vi "SmartMotor_SendCommand - single motor.vi"(0 "VISA In":refnum<visa-resource-name>, 1 "MotorCmd":T4, 2 "Set ModeSelect":T3, 5 "Adhoc Input":T2, 7 "MotorSpecifier(M1)":T1=enum."M1", 9 "ReadWait":u32=50, 11 "error in":errorcluster, 12 "NumericInput":dbl caption="Set Encoder Value(cnts)", 13 "BooleanInput":bool) -> (4 "VISA Out":refnum<visa-resource-name>, 6 "Response Str":string, 8 "Cmd Str out":string, 15 "error out":errorcluster)   [LabVIEW 2020]
doc: "Developed by Kevin Thompson\nkevin@thompsonengineering.net\n\nCopyright 2018-2020\nThompson Engineering, LLC"
uses:
  TD MotorCommands - single motor--enum.ctl
  TD MotorModeSelect_enum.ctl
  TD SerialBusMotorSpecifier_enum.ctl
panel:
  # "Unlisted Command"
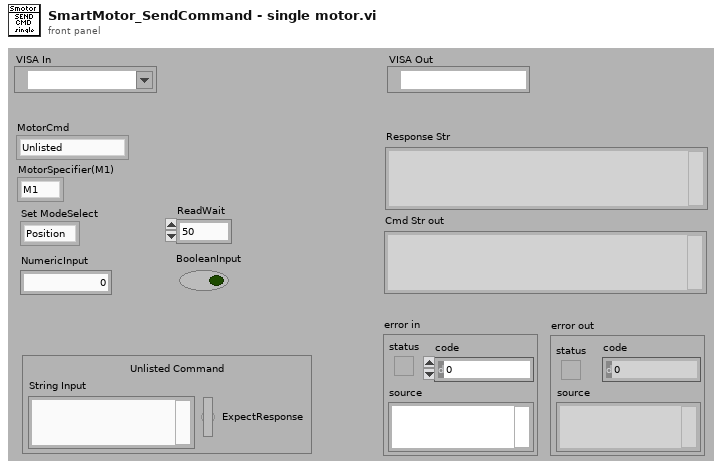
[diagram p1: front panel]
types:
  T1 = typedef "TD SerialBusMotorSpecifier_enum.ctl" = enum16{"None", "Global", "M1", "M2", "M3"}
  T2 = cluster{"String Input":string, "ExpectResponse":bool}
  T3 = typedef "TD MotorModeSelect_enum.ctl" = enum16{"Position", "Velocity", "Torque"}
  T4 = typedef "TD MotorCommands - single motor--enum.ctl" = enum16{"Unlisted", "AbortMotion", "StopMotion", "DisableMotor", "ClearErrors", "ZeroEncoder", "SetMode", "GO", "SetEncoder", "En/Ds LmtSwitchs"}
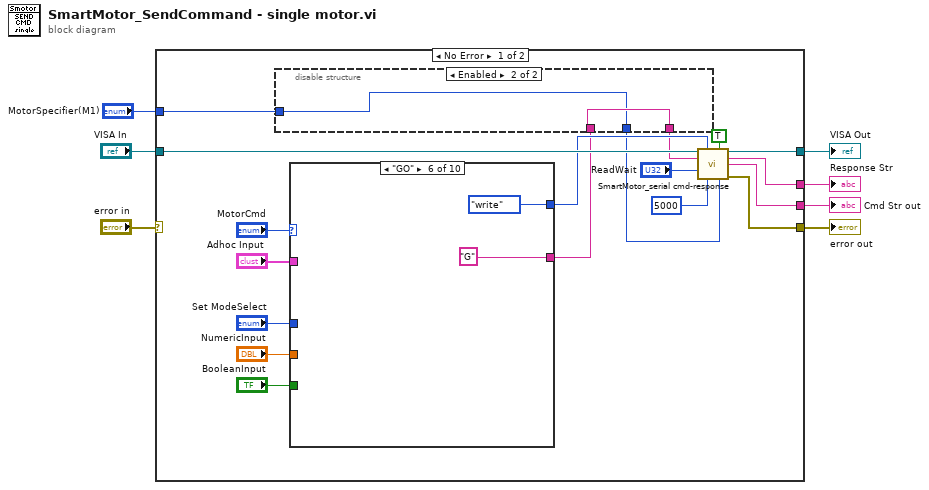
[diagram p0: block diagram]
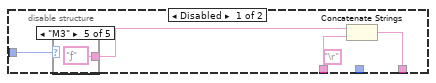
[diagram p2: hidden frame]
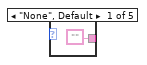
[diagram p3: hidden frame]
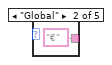
[diagram p4: hidden frame]
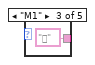
[diagram p5: hidden frame]
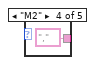
[diagram p6: hidden frame]
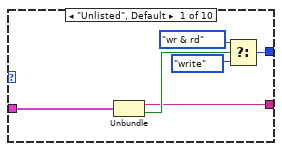
[diagram p7: hidden frame]
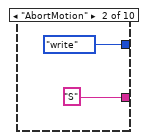
[diagram p8: hidden frame]
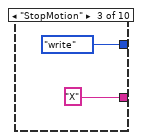
[diagram p9: hidden frame]
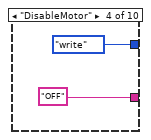
[diagram p10: hidden frame]
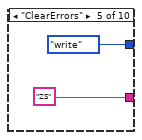
[diagram p11: hidden frame]
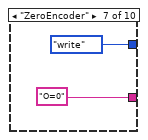
[diagram p12: hidden frame]
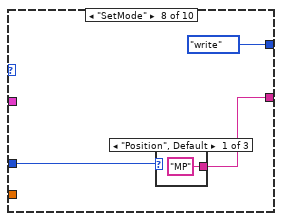
[diagram p13: hidden frame]
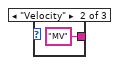
[diagram p14: hidden frame]
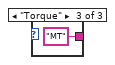
[diagram p15: hidden frame]
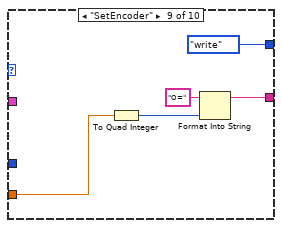
[diagram p16: hidden frame]
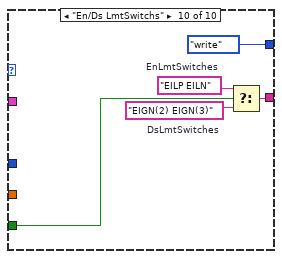
[diagram p17: hidden frame]
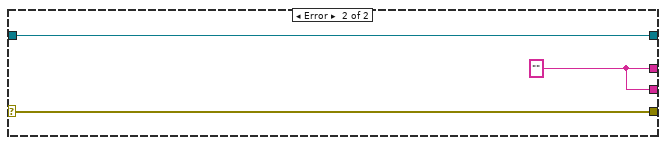
[diagram p18: hidden frame]
diagram:
  n1 = case shown="No Error" "error in" {
    selector: "error in" -> [_ w73]
    tunnel: [w19 w72] -> w7
    tunnel: [w17 w73] -> w6
    tunnel: "VISA In" -> [w20 w72]
    tunnel: [w18 w71] -> w3
    tunnel: [w13 w71] -> w2
    tunnel: "MotorSpecifier(M1)" -> [w12 _]
    frame No Error {
      n2 = case shown="\"GO\"" "MotorCmd" {
        tunnel: "Adhoc Input" -> [w39 _ _ _ _ _ _ _ _ _]
        tunnel: "Set ModeSelect" -> [_ _ _ _ _ _ _ w56 _ _]
        tunnel: "NumericInput" -> [_ _ _ _ _ _ _ _ w62 _]
        tunnel: "BooleanInput" -> [_ _ _ _ _ _ _ _ _ w68]
        tunnel: [w38 enum16{"wr & rd", "write", "read"}."write" ("mode") enum16{"wr & rd", "write", "read"}."write" ("mode") enum16{"wr & rd", "write", "read"}."write" ("mode") enum16{"wr & rd", "write", "read"}."write" ("mode") enum16{"wr & rd", "write", "read"}."write" ("mode") enum16{"wr & rd", "write", "read"}."write" ("mode") enum16{"wr & rd", "write", "read"}."write" ("mode") enum16{"wr & rd", "write", "read"}."write" ("mode") enum16{"wr & rd", "write", "read"}."write" ("mode")] -> w16
        tunnel: [w37 "S" ("cmd") "X" ("cmd") "OFF" ("cmd") "ZS" ("cmd") "G" ("cmd") "O=0" ("cmd") w55 w64 w69] -> w11
        frame "Unlisted", Default {
          n3 = Unbundle(w39) -> ("String Input"=w37:string, "ExpectResponse"=w42:bool)
          n4 = Select(t=enum16{"wr & rd", "write", "read"}."wr & rd" ("mode"), s=w42, f=enum16{"wr & rd", "write", "read"}."write" ("mode")) -> (s? t:f=w38:enum16{"wr & rd", "write", "read"})
        }
        frame "AbortMotion" {
        }
        frame "StopMotion" {
        }
        frame "DisableMotor" {
        }
        frame "ClearErrors" {
        }
        frame "GO" {
        }
        frame "ZeroEncoder" {
        }
        frame "SetMode" {
          n5 = case shown="\"Position\", Default" w56 {
            tunnel: ["MP" "MV" "MT"] -> w55
            frame "Position", Default {
            }
            frame "Velocity" {
            }
            frame "Torque" {
            }
          }
        }
        frame "SetEncoder" {
          n6 = To Quad Integer(1:w62) -> (0:w63:i64)
          n7 = Format Into String(initial string="O=", w63) -> (resulting string=w64:string)  [unwired: 2 in, 1 out]
        }
        frame "En/Ds LmtSwitchs" {
          w66 = "EIGN(2) EIGN(3)"  # DsLmtSwitches
          w67 = "EILP EILN"  # EnLmtSwitches
          n8 = Select(t=w67, s=w68, f=w66) -> (s? t:f=w69:string)
        }
      }
      n9 = disable-structure shown="Enabled" {
        disable-tunnel: w12 -> [w29 w35]
        disable-tunnel: w11 -> [w27 w36]
        disable-tunnel: [w26 w36] -> w10
        disable-tunnel: [_ w35] -> w9
        frame Disabled {
          (unwired) "\r"
          n10 = case shown="\"M3\"" w29 {
            tunnel: ["" "€" "" "‚" "ƒ"] -> w28
            frame "None", Default {
            }
            frame "Global" {
            }
            frame "M1" {
            }
            frame "M2" {
            }
            frame "M3" {
            }
          }
          n11 = Concatenate Strings(w28, w27) -> (w26:string)
        }
        frame Enabled {
        }
      }
      n12 = call "SmartMotor_serial cmd-response.vi"("VISA In"=w20, "mode"=w16, "flush transcvr(F)"=TRUE, "cmd"=w10, "ReadWait"="ReadWait", "Sem Timeout (5000)"=5000 ("Semaphore Timeout"), "MotorSpecifier(None)"=w9) -> ("VISA out"=w19:refnum<visa-resource-name>, "str out"=w18:string, "cmd str out"=w13:string, "error out"=w17:errorcluster)  [unwired: 4 in, 1 out]
    }
    frame Error {
      w71 = "" ("str out")
    }
  }
  "error out" <- w6
  "VISA Out" <- w7
  "Response Str" <- w3
  "Cmd Str out" <- w2
